vi "addData.vi"(8 "error in (no error)":errorcluster, 10 "Data":u8[](array[numeric]), 11 "FrameBuilder in":refnum<class "FrameBuilder.lvclass">) -> (0 "error out":errorcluster, 3 "FrameBuilder out":refnum<class "FrameBuilder.lvclass">)   [LabVIEW 2015, in "FrameBuilder.lvclass"]
uses:
  FrameBuilder.lvclass
  FrameBuilder.lvclass/FrameBuilder.ctl
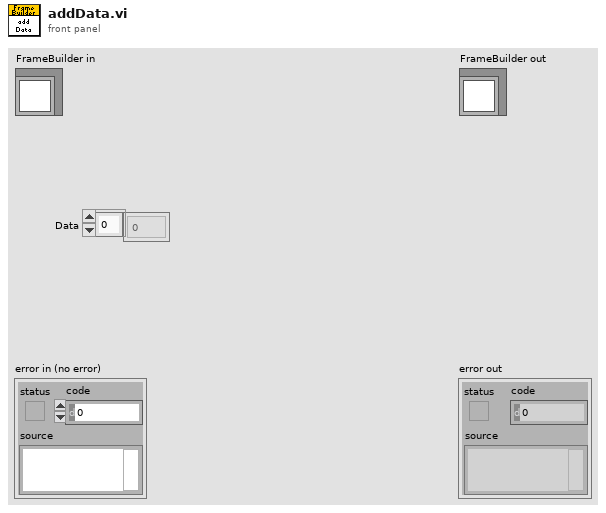
[diagram p1: front panel]
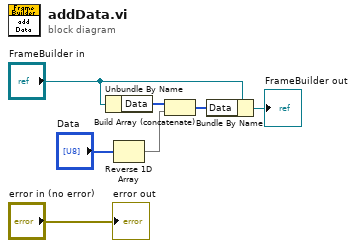
[diagram p0: block diagram]
diagram:
  n1 = Unbundle By Name("FrameBuilder in") -> ("Data"=w5:u8[])
  n2 = Reverse 1D Array(array="Data") -> (reversed array=w2:u8[])
  n3 = Build Array (concatenate)(w5, w2) -> (w4:u8[])
  n4 = Bundle By Name(cluster="FrameBuilder in", "Data"=w4) -> (→"FrameBuilder out":refnum<class "FrameBuilder.lvclass">)
  "error out" <- "error in (no error)"
